vi "Ir sensors time difference.vi"() -> ()   [LabVIEW 2023]
uses:
  <vilib>/DAQmx/read.llb/DAQmx Read (Digital 1D Bool 1Chan 1Samp).vi
  <vilib>/DAQmx/create/channels.llb/DAQmx Create Channel (DI-Digital Input).vi
  <vilib>/DAQmx/miscellaneous.llb/DAQmx Fill In Error Info.vi
panel:
  in  "stop":bool
  in  "lines 2":tag
  in  "lines":tag
  out "Meter":sgl(knob) scale=0.0..150.0
  out "x-y":u32
  # "Speed Meter"
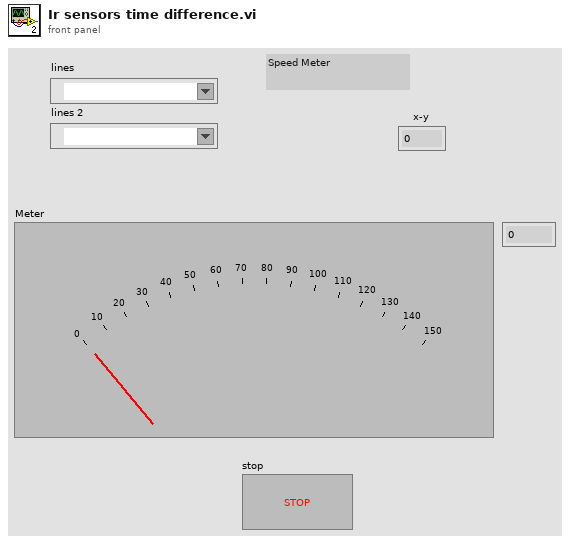
[diagram p1: front panel]
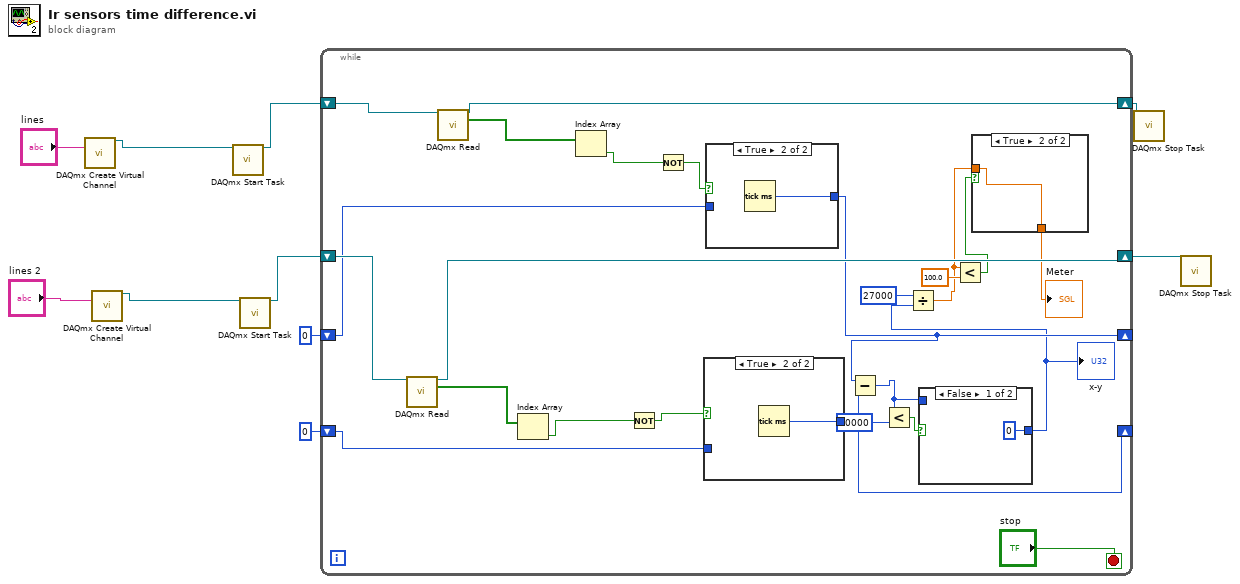
[diagram p0: block diagram]
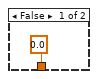
[diagram p2: hidden frame]
diagram:
  n1 = call-poly <vilib>:"DAQmx Create Virtual Channel.vi"("lines"="lines") -> ("task out"=w9:refnum<k21>)  [unwired: 13 in, 1 out]
  n2 = call-poly <vilib>:"DAQmx Create Virtual Channel.vi"("lines"="lines 2") -> ("task out"=w5:refnum<k21>)  [unwired: 13 in, 1 out]
  n3 = call <vilib>:"DAQmx Start Task.vi"("task/channels in"=w9) -> ("task out"=w8:refnum<k21>)  [unwired: 13 in, 1 out]
  n4 = call <vilib>:"DAQmx Start Task.vi"("task/channels in"=w5) -> ("task out"=w4:refnum<k21>)  [unwired: 13 in, 1 out]
  n5 = while {
    shift-right: [w33] -> w7
    shift-left: w8 -> [w34]
    shift-right: [w31] -> w3
    shift-left: w4 -> [w32]
    shift-right: [w24] -> _
    shift-left: u32 0 ("millisecond timer value") -> [w21]
    shift-right: [w23] -> _
    shift-left: u32 0 ("millisecond timer value") -> [w20]
    stop <- "stop" stop-if-true
    n6 = call-poly <vilib>:"DAQmx Read.vi"("task/channels in"=w32) -> ("task out"=w31:refnum<k21>, "data"=w28:bool[])  [unwired: 12 in, 1 out]
    n7 = call-poly <vilib>:"DAQmx Read.vi"("task/channels in"=w34) -> ("task out"=w33:refnum<k21>, "data"=w29:bool[])  [unwired: 12 in, 1 out]
    n8 = Index Array(array=w28) -> (element=w26:bool)  [unwired: 1 in]
    n9 = Index Array(array=w29) -> (element=w27:bool)  [unwired: 1 in]
    n10 = Not(x=w26) -> (.not. x?=w22:bool)
    n11 = Not(x=w27) -> (.not. x?=w25:bool)
    n12 = case shown="True" w22 {
      tunnel: [w39 w40] -> w23
      tunnel: w20 -> [w39 _]
      frame False {
      }
      frame True {
        n13 = Tick Count (ms)() -> (millisecond timer value=w40:u32)
      }
    }
    n14 = case shown="True" w25 {
      tunnel: [w41 w42] -> w24
      tunnel: w21 -> [w41 _]
      frame False {
      }
      frame True {
        n15 = Tick Count (ms)() -> (millisecond timer value=w42:u32)
      }
    }
    n16 = Subtract(x=w24, y=w23) -> (x-y=w17:u32)
    n17 = Less?(x=w17, y=u32 10000) -> (x < y?=w18:bool)
    n18 = case shown="False" w18 {
      tunnel: [u32 0 w38] -> w16
      tunnel: w17 -> [_ w38]
      frame False {
      }
      frame True {
      }
    }
    "x-y" <- w16
    n19 = Divide(x=u32 27000, y=w16) -> (x/y=w12:dbl)
    n20 = Less?(x=w12, y=100.0) -> (x < y?=w13:bool)
    n21 = case shown="True" w13 {
      tunnel: w12 -> [_ w36]
      tunnel: [0.0 w36] -> w11
      frame False {
      }
      frame True {
      }
    }
    "Meter" <- w11
  }
  n22 = call <vilib>:"DAQmx Stop Task.vi"("task/channels in"=w7) -> ()  [unwired: 13 in, 2 out]
  n23 = call <vilib>:"DAQmx Stop Task.vi"("task/channels in"=w3) -> ()  [unwired: 13 in, 2 out]
